vi "isDone.vi"(8 "error in (no error)":errorcluster, 11 "Experiment in":refnum<class "Experiment.lvclass">) -> (0 "error out":errorcluster, 2 "Is done?":bool, 3 "Experiment out":refnum<class "Experiment.lvclass">)   [LabVIEW 2013, in "Experiment.lvclass"]
uses:
  Experiment.lvclass
  Experiment.lvclass/Experiment.ctl
  HSDIO/HSDIO.lvclass
  Analog_output/Analog_Output.lvclass
  DAQmx_pulse_out/DAQmx_pulse_out.lvclass
  Globals.vi
panel:
  out "timeout elapsed?":bool
  out "DAQmx task done?":bool
  out "AO task done?":bool
  out "HSDIO is done?":bool caption="done"
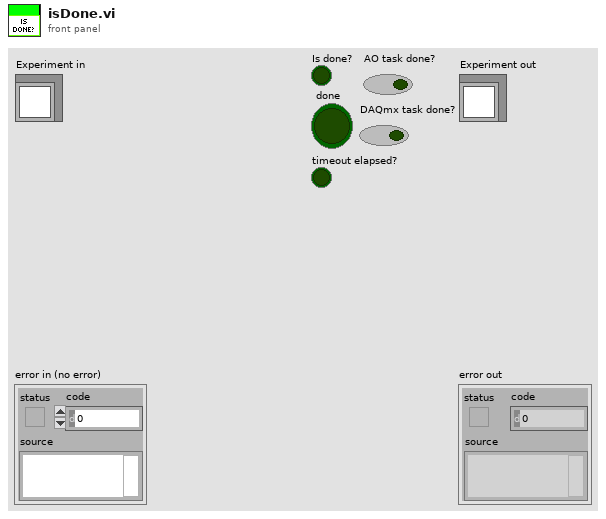
[diagram p1: front panel]
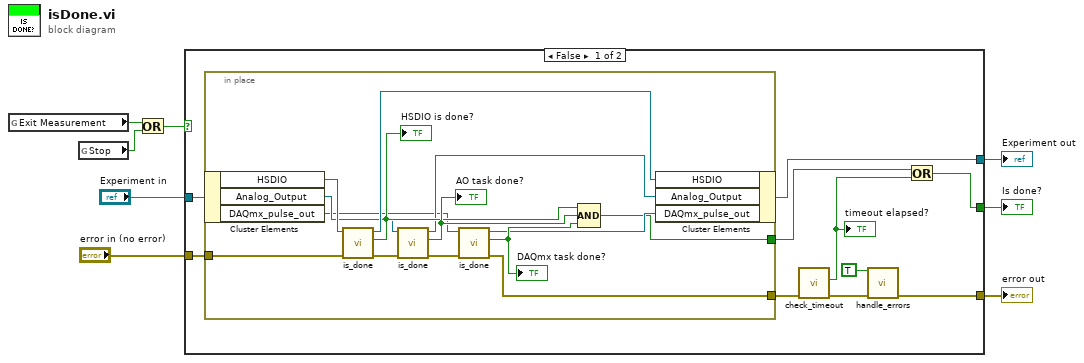
[diagram p0: block diagram]
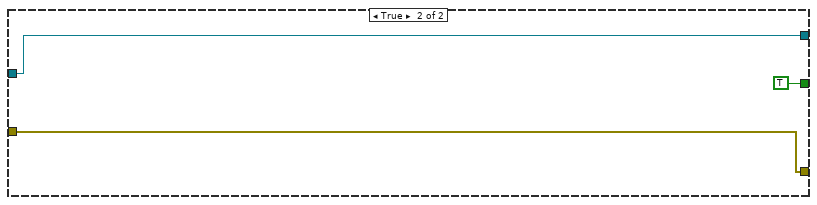
[diagram p2: hidden frame]
diagram:
  n1 = global read "Globals.vi" "Exit Measurement"() -> (w4:bool)
  n2 = global read "Globals.vi" "Stop"() -> (w3:bool)
  n3 = Or(x=w4, y=w3) -> (x .or. y?=w2:bool)
  n4 = case shown="False" w2 {
    tunnel: [w18 w35] -> w8
    tunnel: "error in (no error)" -> [w17 w35]
    tunnel: [w15 w34] -> w6
    tunnel: "Experiment in" -> [w14 w34]
    tunnel: [w10 TRUE] -> w1
    frame False {
      n5 = in-place {
        in-place-border: w17 -> [w21]
        in-place-border: [w20] -> w13
        in-place-border: [w19] -> w11
        n6 = in-place-cluster #1(w14) -> ("HSDIO"=w27:refnum<class "HSDIO.lvclass">, "Analog_Output"=w25:refnum<class "Analog_Output.lvclass">, "DAQmx_pulse_out"=w23:refnum<class "DAQmx_pulse_out.lvclass">)
        n7 = call-dynamic "is_done.vi"("error in (no error)"=w21, "HSDIO in"=w27) -> ("error out"=w28:errorcluster, "HSDIO is done?"=w30:bool, "HSDIO out"=w26:refnum<class "HSDIO.lvclass">)  [unwired: 7 in]
        "HSDIO is done?" <- w30
        n8 = call-dynamic "is_done.vi"("error in (no error)"=w28, "Analog_Output in"=w25) -> ("error out"=w29:errorcluster, "task done?"=w31:bool, "Analog_Output out"=w24:refnum<class "Analog_Output.lvclass">)  [unwired: 7 in]
        "AO task done?" <- w31
        n9 = call-dynamic "is_done.vi"("error in (no error)"=w29, "DAQmx_pulse_out in"=w23) -> ("error out"=w20:errorcluster, "task done?"=w32:bool, "DAQmx_pulse_out out"=w22:refnum<class "DAQmx_pulse_out.lvclass">)  [unwired: 7 in]
        "DAQmx task done?" <- w32
        n10 = Compound Arithmetic op=AND(w30, w31, w32) -> (w19:bool)
        n11 = in-place-cluster #1("HSDIO"=w26, "Analog_Output"=w24, "DAQmx_pulse_out"=w22) -> (w15:refnum<class "Experiment.lvclass">)
      }
      n12 = call "check_timeout.vi"("error in (no error)"=w13) -> ("error out"=w12:errorcluster, "timeout elapsed?"=w9:bool)  [unwired: 8 in, 1 out]
      "timeout elapsed?" <- w9
      n13 = call "handle_errors.vi"("Exit Operation"=TRUE ("Exit Measurement"), "error in (no error)"=w12) -> ("error out"=w18:errorcluster)  [unwired: 13 in]
      n14 = Or(x=w11, y=w9) -> (x .or. y?=w10:bool)
    }
    frame True {
    }
  }
  "error out" <- w8
  "Experiment out" <- w6
  "Is done?" <- w1
